vi "WPI_GyroChannelToAIChannel.vi"(4 "Gyro Channel":T2=enum."AI 1") -> (1 "AI Channel":T1=enum."AI 1")   [LabVIEW 2017]
doc: "This software is licensed. Open the labview\\readme\\WPI Robotics Library Open Source License.txt file for more information."
uses:
  <vilib>/Rock Robotics/SystemInterfaces/AI/FPGA_AIGyroChannel.ctl
  <vilib>/Rock Robotics/SystemInterfaces/AI/FPGA_AIChannel.ctl
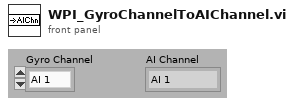
[diagram p1: front panel]
types:
  T1 = typedef "FPGA_AIChannel.ctl" = enum8{"AI 0", "AI 1", "AI 2", "AI 3", "AI MXP 0", "AI MXP 1", "AI MXP 2", "AI MXP 3", "Invalid"}
  T2 = typedef "FPGA_AIGyroChannel.ctl" = enum8{"AI 0", "AI 1", "Invalid"}
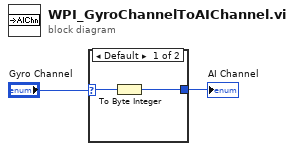
[diagram p0: block diagram]
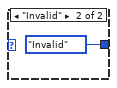
[diagram p2: hidden frame]
diagram:
  n1 = case shown="Default" "Gyro Channel" {
    selector: "Gyro Channel" -> [w4 _]
    tunnel: [w3 FPGA_AIChannel."Invalid" ("AI Channel")] -> w1
    frame Default {
      n2 = To Byte Integer(number=w4) -> (8bit integer=w3:i8)
    }
    frame "Invalid" {
    }
  }
  "AI Channel" <- w1
